vi "Motor_Plus_Impedance_controller_friday.vi"() -> ()   [LabVIEW 2016]
uses:
  <vilib>/Platform/TimedLoop/XDataNode/timing_clust.ctl
  <vilib>/Platform/TimedLoop/XDataNode/nitl_modes.ctl
  <vilib>/Platform/TimedLoop/XDataNode/wakeup.ctl
  <vilib>/Platform/TimedLoop/XDataNode/loadnilvce.vi
  <vilib>/Motion/Express/_s/nimc.ax.power.power.axis.vi
  <vilib>/Motion/Express/_s/nimc.fb.read.readExecutionData.axis.vi
  <vilib>/Motion/Express/_s/nimc.fb.straightLineMove.startStraightLineMove.axis.modeVelocity.0.vi
  <vilib>/Motion/Express/_s/nimc.fb.resetPosition.resetPosition.axis.vi
  <vilib>/Motion/Express/_s/nimc.fb.stopMove.stop.axis.modeDecelerate.vi
  <vilib>/Motion/Express/_s/nimc.ex.power.power.axis.vi
  <vilib>/platform/TimedLoop/XDataNode/XDataNode.xnode
  <vilib>/Motion/BlockNode/FB.NIMotion.xnode
  <vilib>/Platform/TimedLoop/XDataNode/XDNodeRunTimeDep.lvlib
panel:
  out "P_sin x G":dbl=0.25 format="%#_12g"
  out "Torque 2":dbl(knob) scale=-100.0..100.0
  in  "Gravity":dbl format="%#_13g"
  out "post sin":dbl format="%#_13g"
  out "pre sin":dbl format="%#_13g"
  in  "Position 2":dbl=0.25 format="%#_13g"
  out "Adjusted Motor Velocity":dbl format="%.3f"
  out "Adjusted Velocity":dbl(knob) scale=-1.0..1.0
  in  "Reset Position":bool
  in  "Position":dbl=0.25 format="%#_13g"
  in  "Speed":dbl=0.25 format="%#_12g"
  out "Torque":dbl(knob) scale=-5.0..5.0
  out "Position":dbl(knob) scale=-1.0..1.0
  out "Velocity":dbl(knob) scale=-1.0..5.0
  out "Load Cell":dbl(knob) scale=0.0..10.0
  in  "Move to Position?":bool
  out "Load cell, V":dbl format="%.3f"
  out "motor torque, Nm":dbl format="%.3f"
  out "motor velocity, rev/s":dbl format="%.3f"
  out "motor position, rev":dbl format="%.3f"
  in  "STOP VI":bool
  in  "Enable Axis \nControl":bool
  in  "Enable Motor \nDrive":bool
  in  "EMERGENCY MOTOR STOP":bool
  # "Raw Data from System"
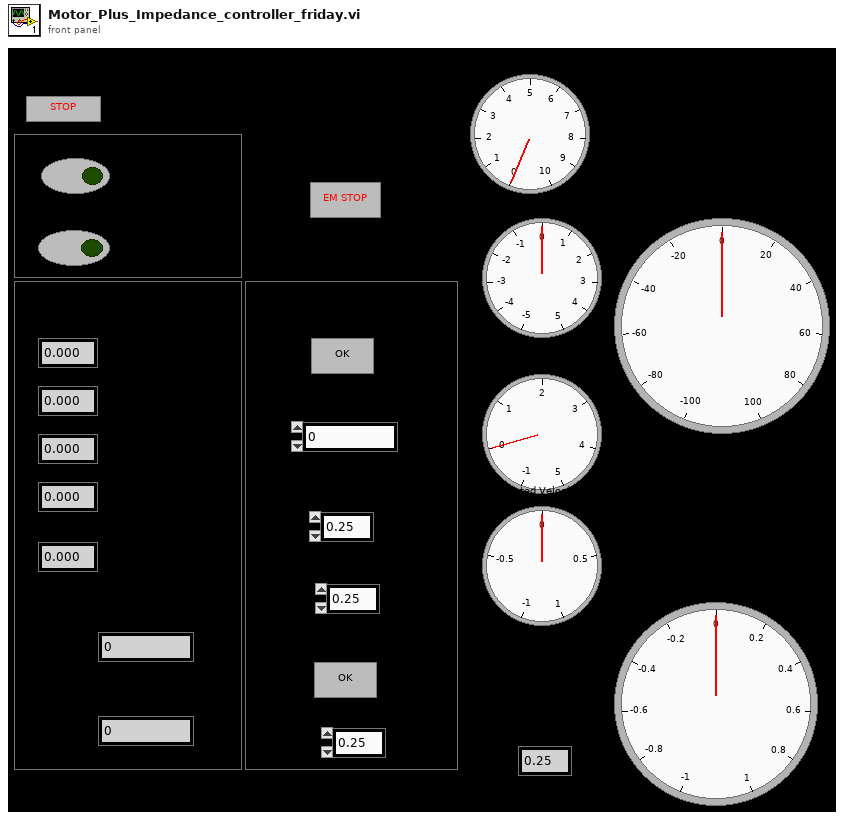
[diagram p1: front panel]
types:
  T1 = typedef "XDNodeRunTimeDep.lvlib/timing_clust.ctl" = cluster{"Expected End [f-1]":u64, "Actual End [f-1]":u64, "Finished Late? [f-1]":bool, "Expected End [i-1]":u64, "Actual End [i-1]":u64, "Finished Late? [i-1]":bool, "Expected Start [i]":u64, "Actual Start [i]":u64, "Expected Start [f]":u64, "Actual Start [f]":u64, "Source Name":string, "Structure Name":string, "Period":i64, "Deadline":i64, "Offset":i64, "Start":i64, "Priority":i32, "Timeout":i32, "Mode":T2, "Wakeup Reason":T3, "Error":errorcluster, "Source Type":string, "Secondary Source Type":string, "Global End Time":u64, "Global Start Time":u64, "Frame Duration":u64, "Iteration Duration":u64, "Assigned CPU":i32, "I/O Scan Engine Mode":u32}
  T2 = typedef "XDNodeRunTimeDep.lvlib/nitl_modes.ctl" = enum32{"No Change", "Process missed periods, maintain original phase", "Discard missed periods, maintain original phase", "Process missed periods, ignore original phase", "Discard missed periods, ignore original phase"}
  T3 = typedef "XDNodeRunTimeDep.lvlib/wakeup.ctl" = enum32{"Normal", "Aborted", "Asynchronous wakeup", "Timing source error", "Timed loop error", "Timeout"}
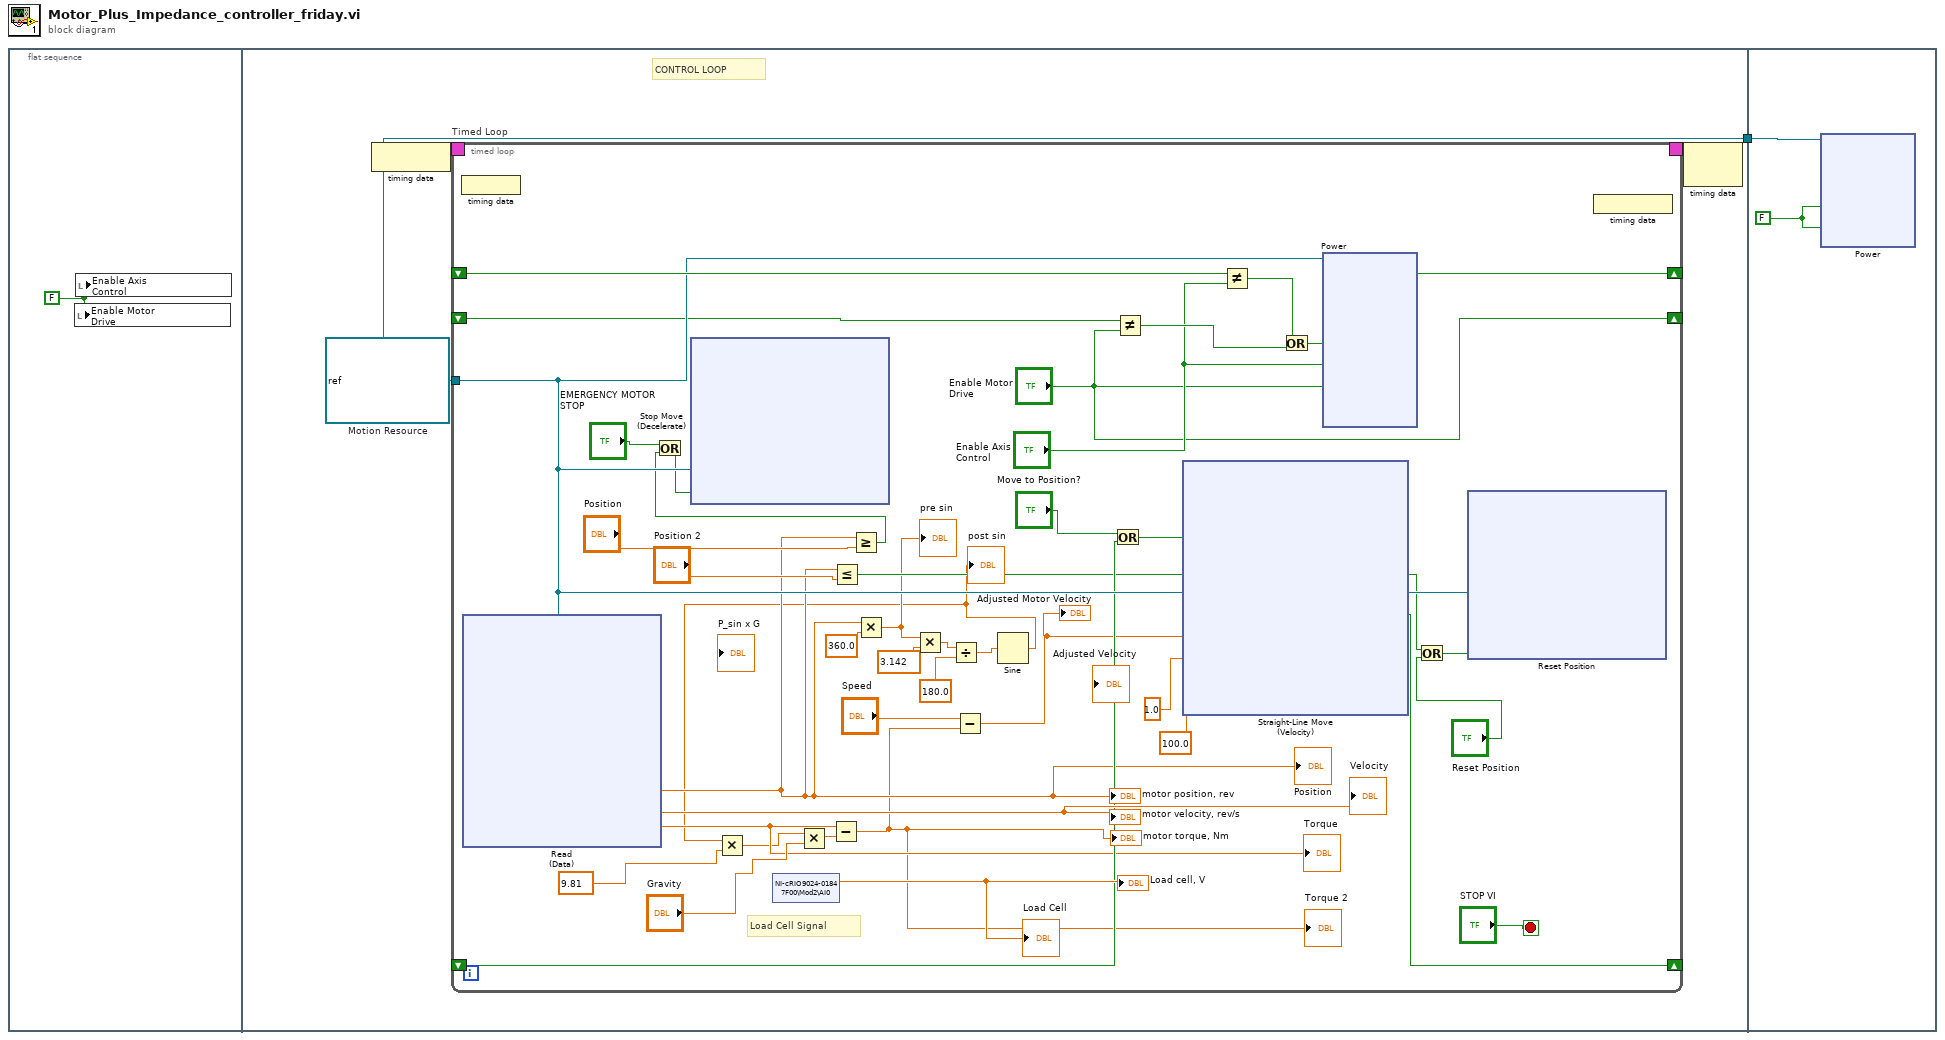
[diagram p0: block diagram]
diagram:
  n1 = flat-sequence {
    tunnel: [w5] -> w1
    tunnel: w1 -> [w125]
    frame #0 {
      w2 = FALSE
      n2 = local write "Enable Motor \nDrive"(w2) -> ()
      n3 = local write "Enable Axis \nControl"(w2) -> ()
    }
    frame #1 {
      w5 = refnum<k21> "nism://NI-cRIO9024-01847F00/Axis 1"  # Motion Resource
      # "CONTROL LOOP"
      n4 = node-c288() -> (w4:T1)
      n5 = timed-loop "Timed Loop" {
        tunnel: w5 -> [w39]
        timing: w4 -> [_]
        timing-out: [_] -> w3
        shift-right: ["Enable Axis \nControl"] -> _
        shift-left: _ -> [w46]
        shift-right: ["Enable Motor \nDrive"] -> _
        shift-left: _ -> [w27]
        shift-right: [w26] -> _
        shift-left: _ -> [w25]
        stop <- "STOP VI" stop-if-true
        # "Load Cell Signal"
        n6 = node-c288() -> ()  [unwired: 1 in]
        n7 = xnode "Read\n(Data)"("resource"=w39) -> ("position"=w20:dbl, "torque"=w16:dbl, "velocity"=→"motor velocity, rev/s" →"Velocity":dbl)  [unwired: 1 in, 3 out]
        "motor position, rev" <- w20
        "Position" <- w20
        "Torque" <- w16
        n8 = shared-variable "NI-cRIO9024-01847F00\\Mod2\\AI0"() -> (→"Load cell, V" →"Load Cell":dbl)  [unwired: 1 in, 1 out]
        n9 = Less Or Equal?(x=w20, y="Position 2") -> (x <= y?=w21:bool)
        n10 = Greater Or Equal?(x=w20, y="Position") -> (x >= y?=w22:bool)
        n11 = Or(x="EMERGENCY MOTOR STOP", y=w22) -> (x .or. y?=w32:bool)
        n12 = xnode "Stop Move\n(Decelerate)"("resource"=w39, "execute"=w32) -> ()  [unwired: 1 in, 3 out]
        n13 = Multiply(x=w20, y=360.0) -> (x*y=w11:dbl)
        "pre sin" <- w11
        n14 = Multiply(x=w11, y=3.142) -> (x*y=w9:dbl)
        n15 = Divide(x=w9, y=180.0) -> (x/y=w8:dbl)
        n16 = Sine(x=w8) -> (sin(x)=w6:dbl)
        "post sin" <- w6
        n17 = Multiply(x=w6, y=9.81) -> (x*y=w13:dbl)
        n18 = Multiply(x=w13, y="Gravity") -> (x*y=w17:dbl)
        n19 = Subtract(x=w16, y=w17) -> (x-y=w14:dbl)
        "motor torque, Nm" <- w14
        "Torque 2" <- w14
        n20 = Subtract(x="Speed", y=w14) -> (x-y=w15:dbl)
        "Adjusted Motor Velocity" <- w15
        n21 = Or(x="Move to Position?", y=w25) -> (x .or. y?=w23:bool)
        n22 = Not Equal?(x=w27, y="Enable Motor \nDrive") -> (x != y?=w44:bool)
        n23 = xnode "Straight-Line Move\n(Velocity)"("resource"=w39, "execute"=w23, "velocity"=w15, "acceleration"=1.0, "deceleration"=100.0) -> ("resource out"=w36:refnum<k21>, "done"=w26:bool)  [unwired: 1 in, 1 out]
        n24 = Not Equal?(x=w46, y="Enable Axis \nControl") -> (x != y?=w45:bool)
        n25 = Or(x=w45, y=w44) -> (x .or. y?=w43:bool)
        n26 = xnode ("Power")("execute"=w43, "enable axis"="Enable Axis \nControl", "enable drive"="Enable Motor \nDrive", "resource"=w39) -> ()  [unwired: 1 in, 6 out]
        n27 = Or(x=w21, y="Reset Position") -> (x .or. y?=w35:bool)
        n28 = xnode "Reset Position"("resource"=w36, "execute"=w35) -> ()  [unwired: 2 in, 3 out]
        n29 = node-c288() -> ()  [unwired: 1 out]
      }
      n30 = node-c288(w3) -> ()  [unwired: 1 out]
    }
    frame #2 {
      w126 = FALSE
      n31 = xnode ("Power")("enable axis"=w126, "enable drive"=w126, "resource"=w125) -> ()  [unwired: 1 in, 2 out]
    }
  }
